vi "Setflex_ray.vi"(8 "error in (no error)":errorcluster, 10 "Set_Val":T1, 11 "OneOfTemplate in":refnum<class "nixnet_grpc_FrameBufferRequest_frame.lvclass">) -> (0 "error out":errorcluster, 3 "OneOfTemplate out":refnum<class "nixnet_grpc_FrameBufferRequest_frame.lvclass">)   [LabVIEW 2019, in "grpc-xnet_client.lvlib" / "nixnet_grpc_FrameBufferRequest_frame.lvclass"]
uses:
  nixnet_grpc_FrameBufferRequest_frame.lvclass
  nixnet_grpc_FrameRequest.ctl
  nixnet_grpc_FrameRequest_type_enum/nixnet_grpc_FrameRequest_type_enum.lvclass
  nixnet_grpc_FrameFlags.ctl
  nixnet_grpc_FrameBufferRequest_frame.lvclass/nixnet_grpc_FrameBufferRequest_frame.ctl
  grpc-xnet_client.lvlib
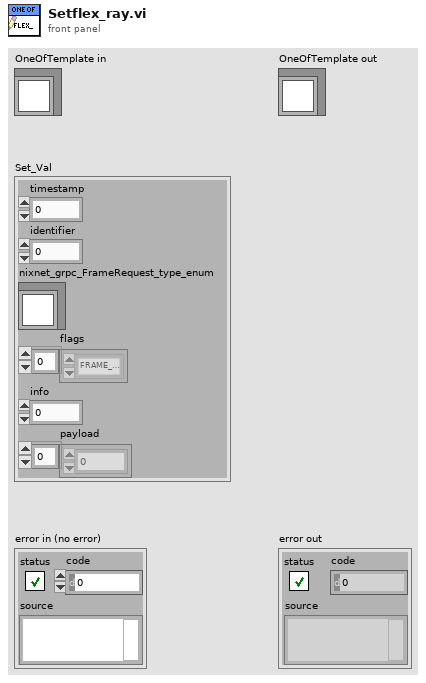
[diagram p1: front panel]
types:
  T1 = typedef "grpc-xnet_client.lvlib/nixnet_grpc_FrameRequest.ctl" = cluster{"timestamp":u64, "identifier":u32, "nixnet_grpc_FrameRequest_type_enum":refnum<class "nixnet_grpc_FrameRequest_type_enum.lvclass">, "flags":T2[], "info":u32, "payload":u8[]}
  T2 = typedef "grpc-xnet_client.lvlib/nixnet_grpc_FrameFlags.ctl" = enum32{"FRAME_FLAGS_UNSPECIFIED", "FRAME_FLAGS_FLEX_RAY_STARTUP", "FRAME_FLAGS_FLEX_RAY_SYNC", "FRAME_FLAGS_FLEX_RAY_PREAMBLE", "FRAME_FLAGS_FLEX_RAY_CH_A", "FRAME_FLAGS_FLEX_RAY_CH_B", "FRAME_FLAGS_LIN_EVENT_SLOT", "FRAME_FLAGS_TRANSMIT_ECHO"}
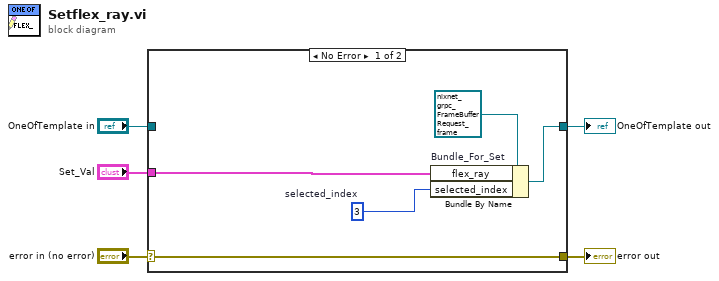
[diagram p0: block diagram]
diagram:
  n1 = case shown="No Error" "error in (no error)" {
    selector: "error in (no error)" -> [w10 w11]
    tunnel: [w10 w11] -> w4
    tunnel: [w9 w12] -> w2
    tunnel: "OneOfTemplate in" -> [_ w12]
    tunnel: "Set_Val" -> [w8 _]
    frame No Error {
      w7 = 3  # selected_index
      n2 = Bundle By Name "Bundle_For_Set"(cluster=refnum<class "nixnet_grpc_FrameBufferRequest_frame.lvclass"> refnum ("OneOfTemplate in"), "flex_ray"=w8, "selected_index"=w7) -> (w9:refnum<class "nixnet_grpc_FrameBufferRequest_frame.lvclass">)
    }
    frame Error {
    }
  }
  "error out" <- w4
  "OneOfTemplate out" <- w2
